vi "ABFLSH_Test.vi"(8 "error in (no error)":errorcluster) -> (0 "error out":errorcluster, 3 "Passed?":bool)   [LabVIEW 2021]
panel:
  out "T":bool
  out "P":bool
  out "Dl":bool
  out "Dv":bool
  out "q":bool
  out "Cp":bool
  out "w":bool
  out "e":bool
  out "s":bool
  out "h":bool
  out "Cv":bool
  out "ierr":bool
  out "D":bool
  out "Inputs":T1={"ab"="TP", "a"=313.5, "b"=632.0, "iflag"=0, "z"=[0.697614699375863, 0.302385300624138]}
  in  "Fluid of interest":string="R410A.MIX"
  out "Outputs":T2 {"s" format="%#_16g"; "Dv" format="%#_16g"; "Dl" format="%#_16g"; "D" format="%#_16g"}
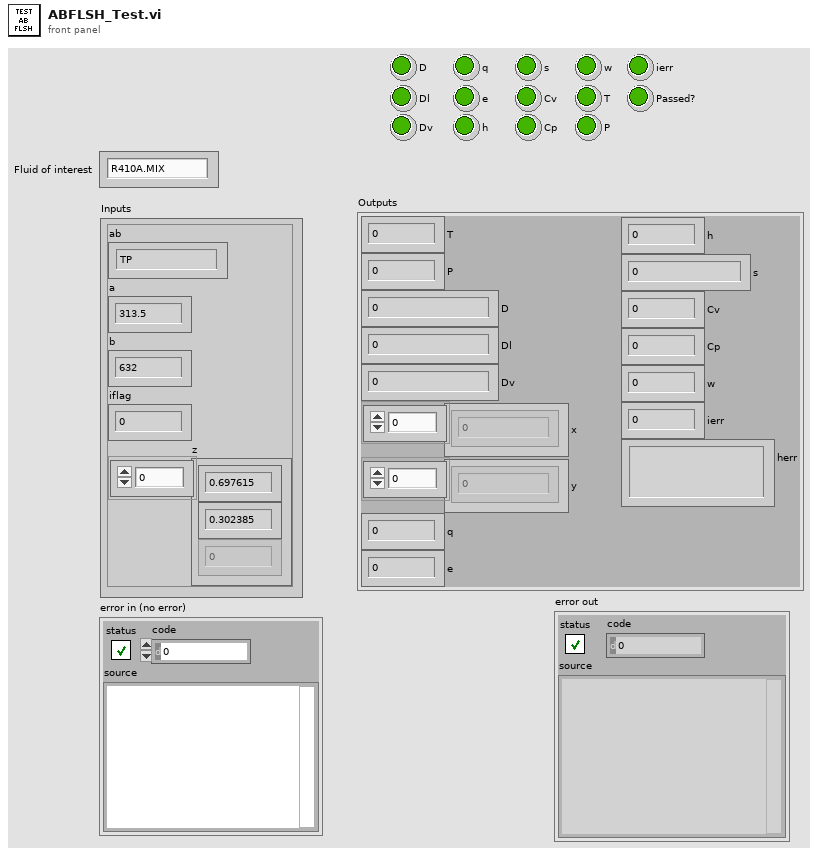
[diagram p1: front panel]
types:
  T1 = cluster{"ab":string, "a":dbl, "b":dbl, "iflag":i32, "z":dbl[]}
  T2 = cluster{"T":dbl, "P":dbl, "D":dbl, "Dl":dbl, "Dv":dbl, "x":dbl[], "y":dbl[], "q":dbl, "e":dbl, "h":dbl, "s":dbl, "Cv":dbl, "Cp":dbl, "w":dbl, "ierr":i32, "herr":string}
  T3 = typedef "Mixture Composition cluster_d.ctl" = cluster{"Mixture Name":string, "Molecular weight (g/mol)":dbl, "Critical temperature (K)":dbl, "Critical Pressure (kPa)":dbl, "Critical Density (mol/L)":dbl, "# Components":i32, "Fluid File Paths":path[], "Component molar fractions":dbl[], "Refprop Main Directory":path, "DLL Version Number":dbl}
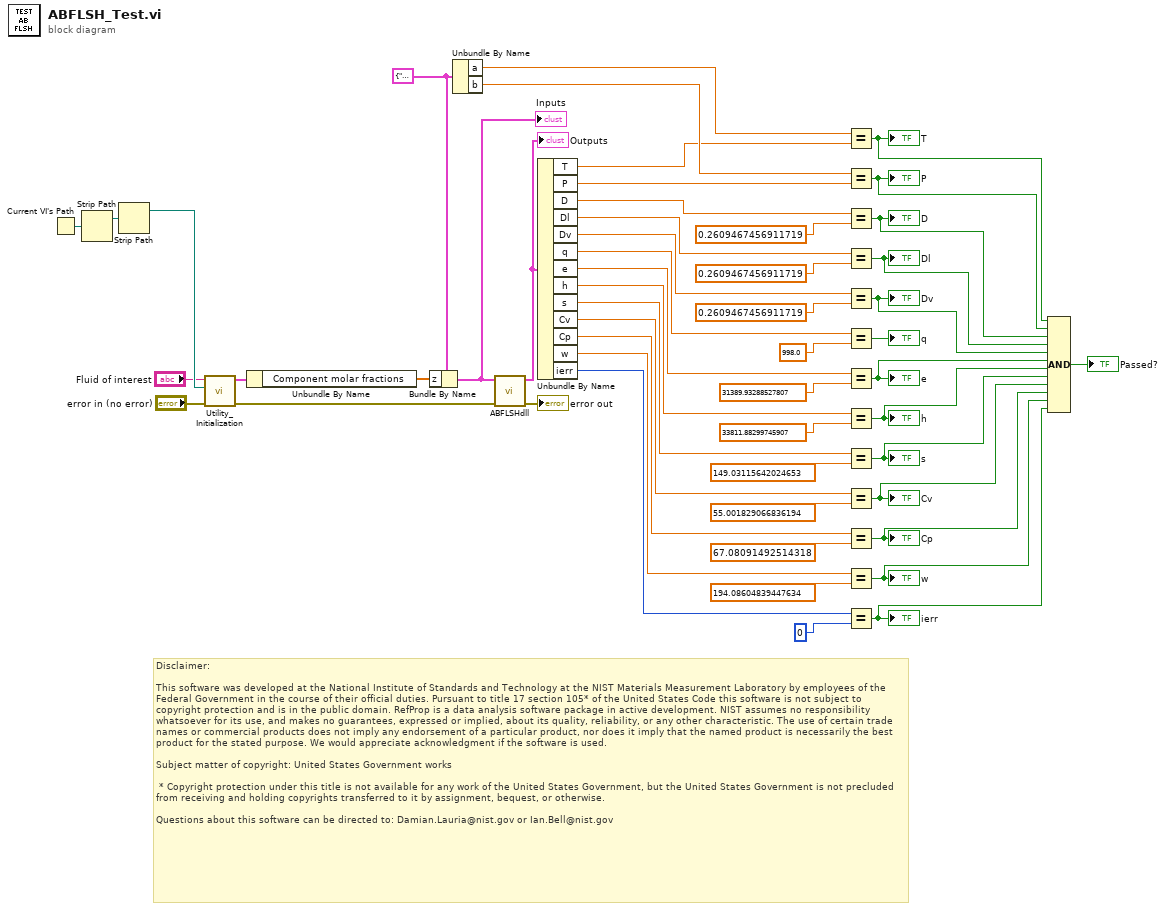
[diagram p0: block diagram]
diagram:
  w49 = T1 {"ab"="TP", "a"=313.5, "b"=632.0, "iflag"=0, "z"=[0.697614699375863, 0.302385300624138, 0.0, 0.0, 0.0, 0.0, 0.0, 0.0, 0.0, 0.0, 0.0, 0.0, 0.0, 0.0, 0.0, 0.0, 0.0, 0.0, 0.0, 0.0]} ("Inputs")
  # "Disclaimer:\n\nThis software was developed at the National Institute of Standards and Technology at the NIST Materials Measurement Laboratory by employees of the Federal Government in the course of their official duties. Pursuant to title 17 section 105* of the United States Code this software is not subject to copyright protection and is in the public domain. RefProp is a data analysis software package in active development. NIST assumes no responsibility whatsoever for its use, and makes no guarantees, expressed or implied, about its quality, reliability, or any other characteristic. The use of certain trade names or commercial products does not imply any endorsement of a particular product, nor does it imply that the named product is necessarily the best product for the stated purpose. We would appreciate acknowledgment if the software is used.\n \nSubject matter of copyright: United States Government works\n  \n * Copyright protection under this title is not available for any work of the United States Government, but the United States Government is not precluded from receiving and holding copyrights transferred to it by assignment, bequest, or otherwise.\n\nQuestions about this software can be directed to: Damian.Lauria@nist.gov or Ian.Bell@nist.gov"
  n1 = Current VI's Path() -> (path=w7:path)
  n2 = Strip Path(path=w7) -> (stripped path=w6:path)  [unwired: 1 out]
  n3 = Strip Path(path=w6) -> (stripped path=w5:path)  [unwired: 1 out]
  n4 = call "Utility_Initialization.vi"("error in (no error)"="error in (no error)", "path"=w5, "Fluidofinterest"="Fluid of interest") -> ("error out"=w10:errorcluster, "Mixure Cluster out"=w3:T3)  [unwired: 6 in, 1 out]
  n5 = Unbundle By Name(w3) -> ("Component molar fractions"=w1:dbl[])
  n6 = Bundle By Name(cluster=w49, "z"=w1) -> (w52:T1)
  "Inputs" <- w52
  n7 = Unbundle By Name(w49) -> ("a"=w8:dbl, "b"=w48:dbl)
  n8 = call "ABFLSHdll.vi"("error in (no error)"=w10, "Inputs"=w52) -> ("error out"=→"error out":errorcluster, "Outputs"=w50:T2)  [unwired: 8 in]
  "Outputs" <- w50
  n9 = Unbundle By Name(w50) -> ("T"=w9:dbl, "P"=w47:dbl, "D"=w31:dbl, "Dl"=w46:dbl, "Dv"=w45:dbl, "q"=w44:dbl, "e"=w43:dbl, "h"=w42:dbl, "s"=w41:dbl, "Cv"=w40:dbl, "Cp"=w39:dbl, "w"=w38:dbl, "ierr"=w37:i32)
  n10 = Equal?(x=w8, y=w9) -> (x = y?=w23:bool)
  "T" <- w23
  n11 = Equal?(x=w48, y=w47) -> (x = y?=w22:bool)
  "P" <- w22
  n12 = Equal?(x=w31, y=0.2609467456911719 ("D")) -> (x = y?=w21:bool)
  "D" <- w21
  n13 = Equal?(x=w46, y=0.2609467456911719 ("Dl")) -> (x = y?=w20:bool)
  "Dl" <- w20
  n14 = Equal?(x=w45, y=0.2609467456911719 ("Dv")) -> (x = y?=w19:bool)
  "Dv" <- w19
  n15 = Equal?(x=w44, y=998.0) -> (x = y?=→"q":bool)
  n16 = Equal?(x=w43, y=31389.93288527807) -> (x = y?=w18:bool)
  "e" <- w18
  n17 = Equal?(x=w42, y=33811.88299745907) -> (x = y?=w17:bool)
  "h" <- w17
  n18 = Equal?(x=w41, y=149.03115642024653 ("s")) -> (x = y?=w16:bool)
  "s" <- w16
  n19 = Equal?(x=w40, y=55.001829066836194 ("Cv")) -> (x = y?=w15:bool)
  "Cv" <- w15
  n20 = Equal?(x=w39, y=67.08091492514318 ("Cp")) -> (x = y?=w14:bool)
  "Cp" <- w14
  n21 = Equal?(x=w38, y=194.08604839447634 ("w")) -> (x = y?=w13:bool)
  "w" <- w13
  n22 = Equal?(x=w37, y=0) -> (x = y?=w12:bool)
  "ierr" <- w12
  n23 = Compound Arithmetic op=AND(w23, w22, w21, w20, w19, w18, w17, w16, w15, w14, w13, w12) -> (→"Passed?":bool)
